vi "Offset Inline Buffers.vi"(8 "error in (no error)":errorcluster, 10 "base Inline Buffer":refnum<class "Buffer.lvclass">, 11 "Framework in":refnum<class "Framework.lvclass">) -> (0 "error out":errorcluster, 3 "Framework out":refnum<class "Framework.lvclass">)   [LabVIEW 2019, in "DSF Core.lvlib" / "Framework.lvclass"]
uses:
  Framework.lvclass
  Buffer/Buffer.lvclass
  C:/Program Files (x86)/National Instruments/LabVIEW 2019/vi.lib/NI/Memory Manager/Classes/Pointer/Pointer.lvclass
  Framework.lvclass/Framework.ctl
  Plugin/Plugin.lvclass/Plugin.ctl
  Transfer Group/Transfer Group.lvclass/Transfer Group.ctl
  Buffers/Buffers.lvclass/Buffers.ctl
  <vilib>/NI/Memory Manager/Classes/Pointer/Pointer.lvclass/Pointer.ctl
  Buffer/Buffer.lvclass/Buffer.ctl
  Transfer/Transfer.lvclass/Transfer.ctl
  Transfer Group/Align Buffers.vi
  Transfer/Align Buffers.vi
  Buffers/Align Inline Buffer.vi
  Buffers/Align Buffers.vi
  Buffer/Align to Base Buffer.vi
  <vilib>/NI/Memory Manager/Classes/Pointer/Get Address.vi
  <vilib>/NI/Memory Manager/Classes/Pointer/Encapsulate.vi
  <vilib>/NI/Memory Manager/Classes/Pointer/Get Size.vi
  <vilib>/NI/Memory Manager/Classes/Pointer/Is Null.vi
  <vilib>/NI/Memory Manager/Classes/Pointer/Set Size.vi
  <vilib>/NI/Memory Manager/Classes/Pointer/Set Address.vi
  <vilib>/NI/Memory Manager/Classes/Pointer/Check Null Pointer.vi
  <vilib>/NI/Memory Manager/Classes/Pointer/Set Internal.vi
  <vilib>/NI/Memory Manager/Classes/Pointer/Errors.vi
  <vilib>/NI/Memory Manager/Classes/Pointer/Null Pointer.vi
  <vilib>/NI/Memory Manager/Classes/Pointer/Create Error.vi
  <vilib>/NI/Memory Manager/VIs/New Error Cluster.vi
  <vilib>/NI/Memory Manager/VIs/New Error Cluster (512B).vi
  <vilib>/NI/Memory Manager/VIs/Set Error Status.vi
  <vilib>/NI/Memory Manager/VIs/Set Error Code.vi
  <vilib>/NI/Memory Manager/VIs/Set Error Source.vi
  <vilib>/NI/Memory Manager/Constants/Constants.vi
  <vilib>/NI/Memory Manager/Constants/Library Name.vi
  <vilib>/NI/Memory Manager/Classes/Pointer/Pointer Error Info.vi
  <vilib>/NI/Memory Manager/VIs/Write String to Source.vi
  <vilib>/NI/Memory Manager/Constants/Pointer Class Name.vi
  Plugin/Plugin.lvclass
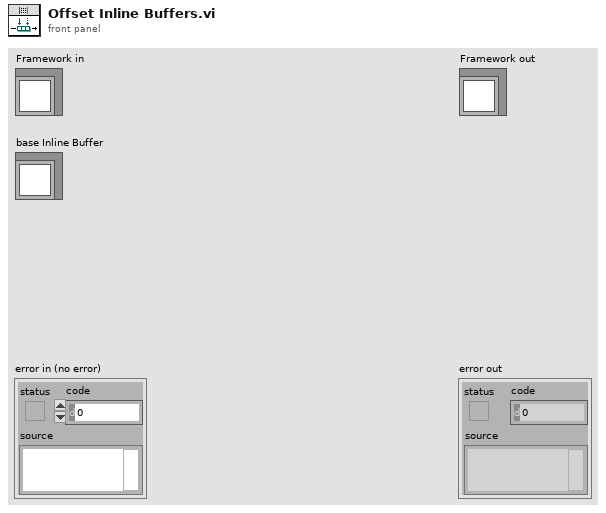
[diagram p1: front panel]
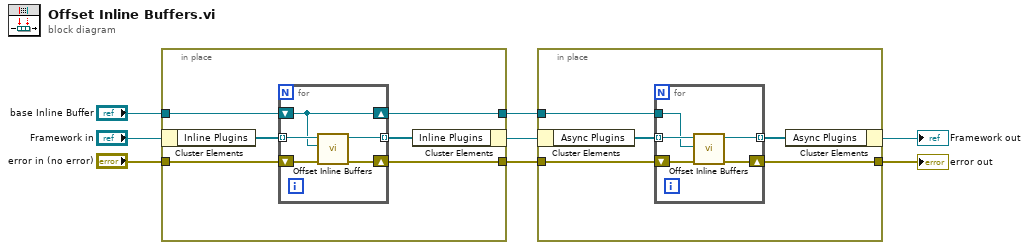
[diagram p0: block diagram]
diagram:
  n1 = in-place {
    in-place-border: "error in (no error)" -> [w11]
    in-place-border: [w12] -> w7
    in-place-border: "base Inline Buffer" -> [w10]
    in-place-border: [w9] -> w2
    n2 = in-place-cluster #1("Framework in") -> ("Inline Plugins"=w14:refnum<class "Plugin.lvclass">[])
    n3 = for {
      tunnel: w14 -> [w19] mode=indexing
      tunnel: [w18] -> w13 mode=indexing
      shift-right: [w17] -> w12
      shift-left: w11 -> [w16]
      shift-right: [w15] -> w9
      shift-left: w10 -> [w15]
      n4 = call "Offset Inline Buffers.vi"("error in (no error)"=w16, "base Inline Buffer"=w15, "Plugin in"=w19) -> ("error out"=w17:errorcluster, "Plugin out"=w18:refnum<class "Plugin.lvclass">)  [unwired: 7 in]
    }
    n5 = in-place-cluster #1("Inline Plugins"=w13) -> (w3:refnum<class "Framework.lvclass">)
  }
  n6 = in-place {
    in-place-border: w7 -> [w21]
    in-place-border: [w22] -> w5
    in-place-border: w2 -> [w20]
    n7 = in-place-cluster #2(w3) -> ("Async Plugins"=w24:refnum<class "Plugin.lvclass">[])
    n8 = for {
      tunnel: w24 -> [w29] mode=indexing
      tunnel: [w28] -> w23 mode=indexing
      shift-right: [w27] -> w22
      shift-left: w21 -> [w26]
      tunnel: w20 -> [w25]
      n9 = call "Offset Inline Buffers.vi"("error in (no error)"=w26, "base Inline Buffer"=w25, "Plugin in"=w29) -> ("error out"=w27:errorcluster, "Plugin out"=w28:refnum<class "Plugin.lvclass">)  [unwired: 7 in]
    }
    n10 = in-place-cluster #2("Async Plugins"=w23) -> (→"Framework out":refnum<class "Framework.lvclass">)
  }
  "error out" <- w5
